vi "g_Sol OutputsALB.vi"(7 "Action":enum16{"initialize", "read", "write"}(ring), 9 "Solenoid in":T1, 11 "Parameter":T2) -> (2 "DI out":T3)   [LabVIEW 2017]
uses:
  CtrlRefs/SolenoidsDisplayALB.ctl
  CtrlRefs/SolenoidsALB.ctl
  <vilib>/Rock Robotics/WPI/Solenoid/WPI_SolenoidValue.ctl
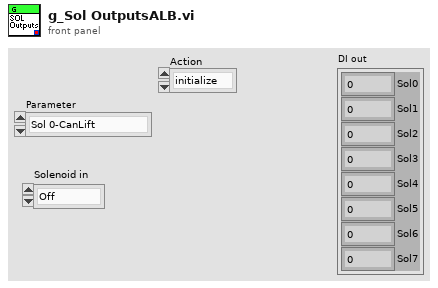
[diagram p1: front panel]
types:
  T1 = typedef "WPI_SolenoidValue.ctl" = enum16{"Off", "On", "Forward", "Reverse"}
  T2 = typedef "SolenoidsALB.ctl" = enum16{"Sol 0-CanLift", "Sol1- StackLiftUp", "Sol2- StackLiftDn", "Sol3- CanPosition", "Sol4- CanLift4", "Sol5- CanLift5", "Sol6- Latch1", "Sol7- Latch2"}
  T3 = typedef "SolenoidsDisplayALB.ctl" = cluster{"CanLift (0)":i32, "StackLift1 (1)":i32, "StackLift2 (2)":i32, "CanPosition (3)":i32, "CanLift4 (4)":i32, "CanLift (5)":i32, "Latch1 (6)":i32, "Latch2 (7)":i32}
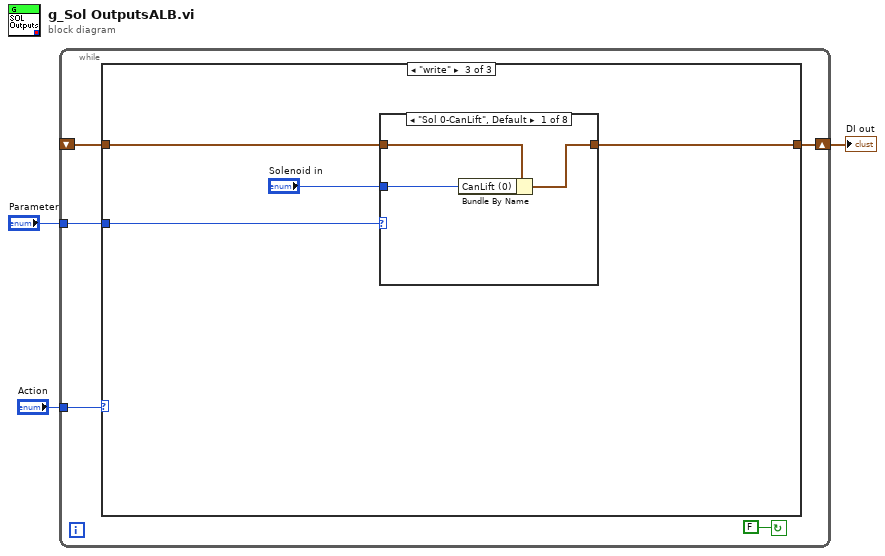
[diagram p0: block diagram]
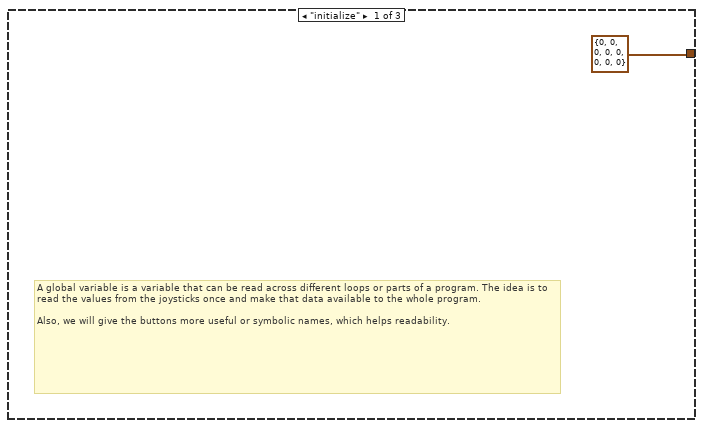
[diagram p2: hidden frame]
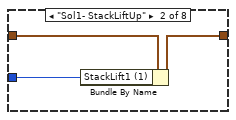
[diagram p4: hidden frame]
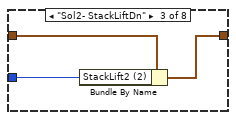
[diagram p5: hidden frame]
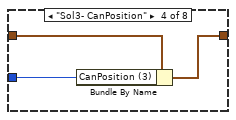
[diagram p6: hidden frame]
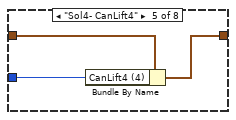
[diagram p7: hidden frame]
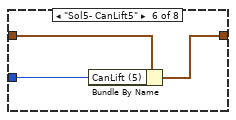
[diagram p8: hidden frame]
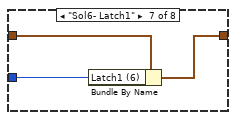
[diagram p9: hidden frame]
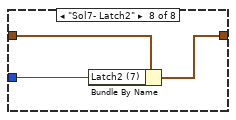
[diagram p10: hidden frame]
diagram:
  n1 = while {
    tunnel: "Action" -> [w7]
    shift-right: [w6] -> w1
    shift-left: _ -> [w5]
    tunnel: "Parameter" -> [w4]
    stop <- FALSE continue-if-true
    n2 = case shown="\"write\"" w7 {
      tunnel: [T3 {"CanLift (0)"=0, "StackLift1 (1)"=0, "StackLift2 (2)"=0, "CanPosition (3)"=0, "CanLift4 (4)"=0, "CanLift (5)"=0, "Latch1 (6)"=0, "Latch2 (7)"=0} ("DI out") w10 w13] -> w6
      tunnel: w5 -> [_ w10 w14]
      tunnel: w4 -> [_ _ w12]
      frame "initialize" {
        # "A global variable is a variable that can be read across different loops or parts of a program. The idea is to read the values from the joysticks once and make that data available to the whole program.\n \nAlso, we will give the buttons more useful or symbolic names, which helps readability."
      }
      frame "read", Default {
      }
      frame "write" {
        n3 = case shown="\"Sol 0-CanLift\", Default" w12 {
          tunnel: "Solenoid in" -> [w15 w18 w21 w24 w27 w30 w33 w36]
          tunnel: w14 -> [w17 w20 w23 w26 w29 w32 w35 w38]
          tunnel: [w16 w19 w22 w25 w28 w31 w34 w37] -> w13
          frame "Sol 0-CanLift", Default {
            n4 = Bundle By Name(cluster=w17, "CanLift (0)"=w15) -> (w16:T3)
          }
          frame "Sol1- StackLiftUp" {
            n5 = Bundle By Name(cluster=w20, "StackLift1 (1)"=w18) -> (w19:T3)
          }
          frame "Sol2- StackLiftDn" {
            n6 = Bundle By Name(cluster=w23, "StackLift2 (2)"=w21) -> (w22:T3)
          }
          frame "Sol3- CanPosition" {
            n7 = Bundle By Name(cluster=w26, "CanPosition (3)"=w24) -> (w25:T3)
          }
          frame "Sol4- CanLift4" {
            n8 = Bundle By Name(cluster=w29, "CanLift4 (4)"=w27) -> (w28:T3)
          }
          frame "Sol5- CanLift5" {
            n9 = Bundle By Name(cluster=w32, "CanLift (5)"=w30) -> (w31:T3)
          }
          frame "Sol6- Latch1" {
            n10 = Bundle By Name(cluster=w35, "Latch1 (6)"=w33) -> (w34:T3)
          }
          frame "Sol7- Latch2" {
            n11 = Bundle By Name(cluster=w38, "Latch2 (7)"=w36) -> (w37:T3)
          }
        }
      }
    }
  }
  "DI out" <- w1
